vi "ADC_select_primary.vi"(11 "ADC-primary-select":i16(ring) items=["Mod2/AI0", "Mod2/AI1", "Mod2/AI2", "Mod2/AI3", ""]) -> (2 "ADC-all":fxp<+/-,24,5>[](array[numeric]), 3 "Primary-ADC":fxp<+/-,24,5>)   [LabVIEW 2017]
uses:
  <vilib>/rvi/eio/common/nirviEmuTemplateMethod_errors.vi
  <vilib>/eio/EIONode/EIONode.xnode
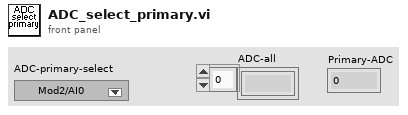
[diagram p1: front panel]
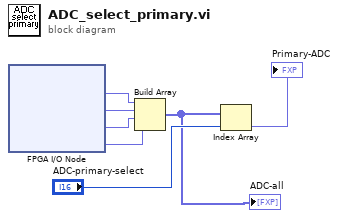
[diagram p0: block diagram]
diagram:
  n1 = xnode "FPGA I/O Node"() -> ("Mod2/AI0"=w4:fxp<+/-,24,5>, "Mod2/AI1"=w5:fxp<+/-,24,5>, "Mod2/AI2"=w6:fxp<+/-,24,5>, "Mod2/AI3"=w7:fxp<+/-,24,5>)  [unwired: 4 in, 4 out]
  n2 = Build Array(w4, w5, w6, w7) -> (w1:fxp<+/-,24,5>[])
  "ADC-all" <- w1
  n3 = Index Array(array=w1, index="ADC-primary-select") -> (element=→"Primary-ADC":fxp<+/-,24,5>)
